vi "Get VI Settings - Method Options - Front Panels.vi"(8 "error in (no error)":errorcluster {"code" format="Error %.0f"}, 11 "VIDoc Printer In":refnum<class "VIDoc Printer.lvclass">) -> (0 "error out":errorcluster {"code" format="Error %.0f"}, 2 "Front Panels":bool=TRUE, 3 "VIDoc Printer Out":refnum<class "VIDoc Printer.lvclass">)   [LabVIEW 2023, in "VIDoc Printer.lvlib" / "VIDoc Printer.lvclass"]
uses:
  VIDoc Printer.lvclass
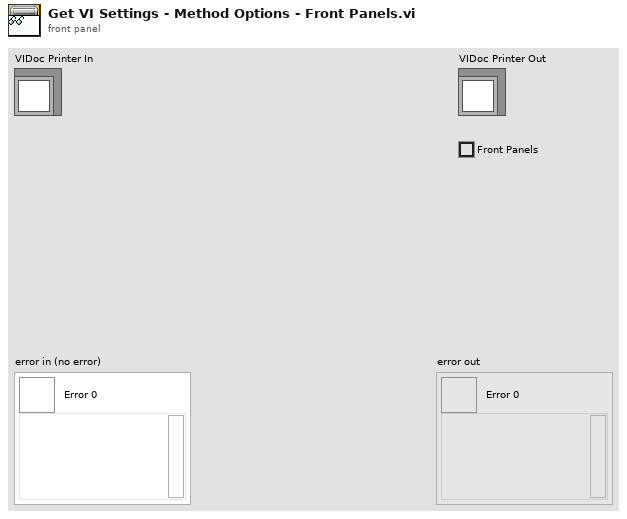
[diagram p1: front panel]
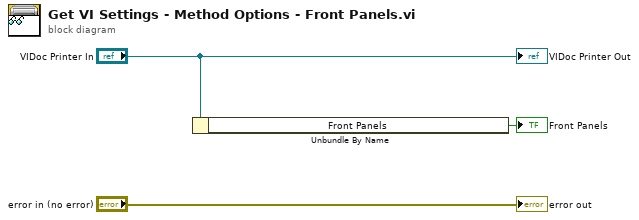
[diagram p0: block diagram]
diagram:
  n1 = Unbundle By Name("VIDoc Printer In") -> ("Front Panels"=→"Front Panels":bool)
  "error out" <- "error in (no error)"
  "VIDoc Printer Out" <- "VIDoc Printer In"
